vi "AVI-Bundle playback parameters.vi"(9 "Fill time":dbl, 10 "TIME SERIES":T1 {"Basic Image meta data"."Frame Size" items=["100X100"=100, "128X128"=128, "200X200"=200, "256X256"=256, "512X512"=512, "1024x1024"=1024, "2048x2048"=2048]}, 11 "I16 image ref":T4) -> (3 "AVI playback header info cluster":T5)   [LabVIEW 2017]
uses:
  Typedefs/AVI playback header info cluster.ctl
  <vilib>/vision/Image Controls.llb/IMAQ Image.ctl
  Functional Imaging Viewer/SubVIs/Experiment header interface/Typedefs/Header subclusters/Header params-Time Series.ctl
  Functional Imaging Viewer/SubVIs/Experiment header interface/Typedefs/Header subclusters/Header params-Basic image meta data.ctl
  Typedefs/Frame Size.ctl
  Global Variables/General Globals.vi
  <resource>/objmgr/IMAQImage.rc
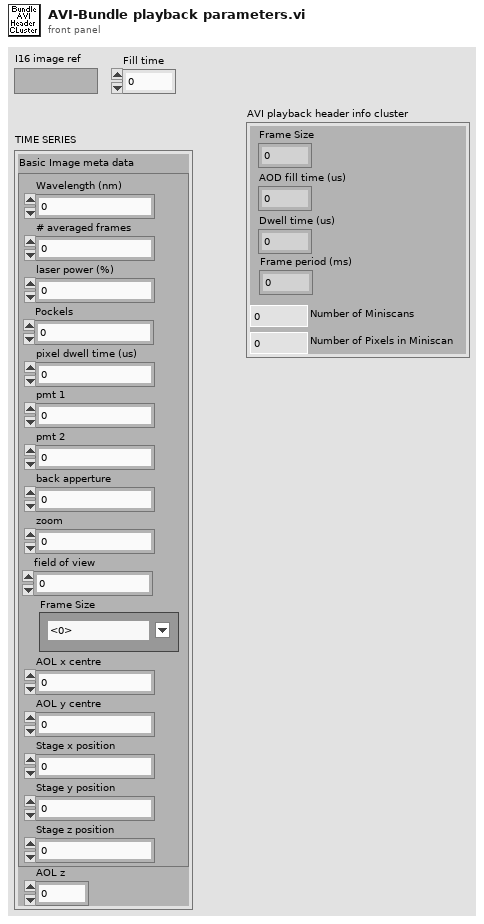
[diagram p1: front panel]
types:
  T1 = typedef "Header params-Time Series.ctl" = cluster{"Basic Image meta data":T2, "AOL z":dbl}
  T2 = typedef "Header params-Basic image meta data.ctl" = cluster{"Wavelength (nm)":dbl, "# averaged frames":dbl, "laser power (%)":dbl, "Pockels":dbl, "pixel dwell time (us)":dbl, "pmt 1":dbl, "pmt 2":dbl, "back apperture":dbl, "zoom":dbl, "field of view":dbl, "Frame Size":T3, "AOL x centre":dbl, "AOL y centre":dbl, "Stage x position":dbl, "Stage y position":dbl, "Stage z position":dbl}
  T3 = typedef "Frame Size.ctl" = u16
  T4 = typedef "IMAQ Image.ctl" = refnum<image>
  T5 = typedef "AVI playback header info cluster.ctl" = cluster{"Frame Size":u32, "AOD fill time (us)":dbl, "Dwell time (us)":dbl, "Frame period (ms)":dbl, "Number of Miniscans":u16, "Number of Pixels in Miniscan":u16}
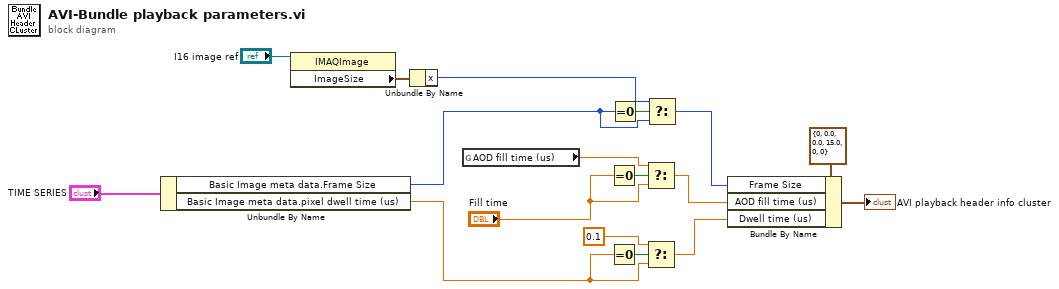
[diagram p0: block diagram]
diagram:
  n1 = Unbundle By Name("TIME SERIES") -> ("Basic Image meta data.Frame Size"=w9:T3, "Basic Image meta data.pixel dwell time (us)"=w5:dbl)
  n2 = property class="IMAQImage"(reference="I16 image ref") -> ("ImageSize"=w12:cluster{"x":i32, "y":i32})  [unwired: 1 in, 2 out]
  n3 = Unbundle By Name(w12) -> ("x"=w7:i32)
  n4 = global read "General Globals.vi" "AOD fill time (us)"() -> (w16:dbl)
  n5 = Equal To 0?(x="Fill time") -> (x = 0?=w14:bool)
  n6 = Equal To 0?(x=w5) -> (x = 0?=w6:bool)
  n7 = Equal To 0?(x=w9) -> (x = 0?=w10:bool)
  n8 = Select(t=w16, s=w14, f="Fill time") -> (s? t:f=w15:dbl)
  n9 = Select(t=0.1 ("Dwell time (us)"), s=w6, f=w5) -> (s? t:f=w4:dbl)
  n10 = Select(t=w7, s=w10, f=w9) -> (s? t:f=w8:i32)
  n11 = Bundle By Name(cluster=T5 {"Frame Size"=0, "AOD fill time (us)"=0.0, "Dwell time (us)"=0.0, "Frame period (ms)"=15.0, "Number of Miniscans"=0, "Number of Pixels in Miniscan"=0} ("AVI playback header info cluster"), "Frame Size"=w8, "AOD fill time (us)"=w15, "Dwell time (us)"=w4) -> (→"AVI playback header info cluster":T5)
